vi "Polling Core.vi"(8 "Error In":errorcluster, 11 "LS218 in":refnum<class "LS218.lvclass">) -> (0 "Error Out":errorcluster, 3 "LS218 out":refnum<class "LS218.lvclass">)   [LabVIEW 2015, in "LS218.lvlib" / "LS218.lvclass"]
doc: "Implement the pseudo-periodic action here."
uses:
  LS218.lvclass
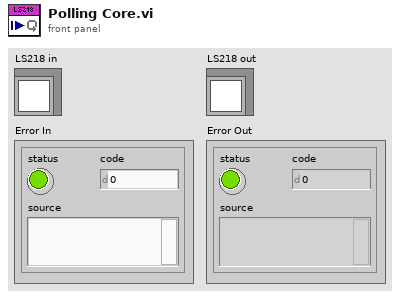
[diagram p1: front panel]
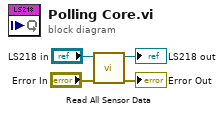
[diagram p0: block diagram]
diagram:
  n1 = call "Read All Sensor Data.vi"("error in (no error)"="Error In", "LS218 in"="LS218 in") -> ("error out"=→"Error Out":errorcluster, "LS218 out"=→"LS218 out":refnum<class "LS218.lvclass">)  [unwired: 8 in]
